vi "MeasureVoltage.vi"(8 "error in (no error)":errorcluster, 11 "DMMArray in":refnum<class "DMMArray.lvclass">) -> (0 "error out":errorcluster, 3 "DMMArray out":refnum<class "DMMArray.lvclass">)   [LabVIEW 2020, in "DMMArray.lvclass"]
uses:
  DMMArray/DMMArray.lvclass
  IReference/IDMM.lvclass
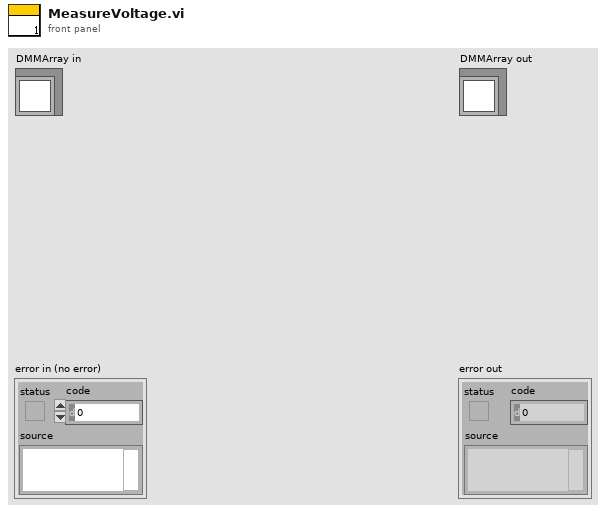
[diagram p1: front panel]
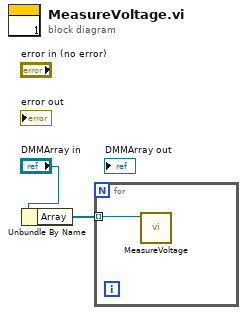
[diagram p0: block diagram]
diagram:
  n1 = Unbundle By Name("DMMArray in") -> ("Array"=w1:refnum<class "IDMM.lvclass">[])
  n2 = for {
    tunnel: w1 -> [w3] mode=indexing
    n3 = call-dynamic "MeasureVoltage.vi"("IDMM in"=w3) -> ()  [unwired: 9 in, 2 out]
  }
